vi "LoadConfig.vi"(10 "Path":string, 11 "PN":string) -> (3 "Cluster":T1 {"Screw 2" items=["0", "1", "2", "3", "4", "5", "6", "7", "8", "9", "10", "11", "12", "13", "14", "15", "16", "17", "18", "19", "20", "21", "22", "23", "24", "25", "26", "27", "28", "29", "30"]; "M6_Camera" items=["0", "1", "2", "3", "4", "5", "6", "7", "8", "9", "10", "11", "12", "13", "14", "15", "16", "17", "18", "19", "20", "21", "22", "23", "24", "25", "26", "27", "28", "29", "30"]; "L/R" items=["NA", "RHC-VAC", "RHD-HVAC", "LHD-VAC", "LHD-HVAC", ""]})   [LabVIEW 2020]
uses:
  NewPNConfig.ctl
  <vilib>/Utility/config.llb/Read Key (String).vi
  <vilib>/Utility/config.llb/Read Key (I32).vi
  <vilib>/Utility/config.llb/NI_LVConfig.lvlib
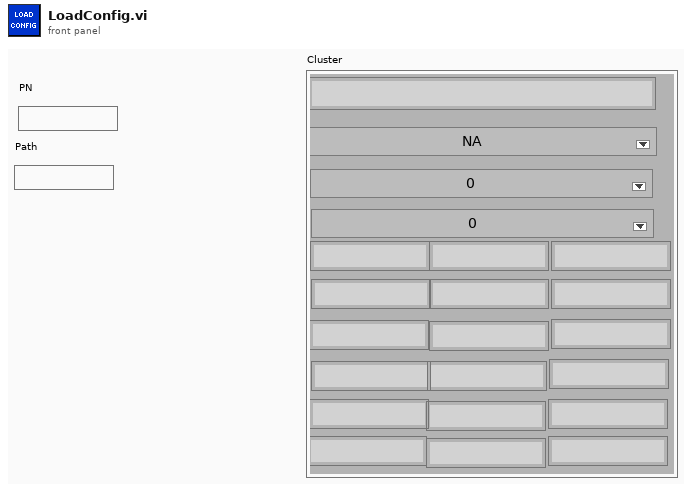
[diagram p1: front panel]
types:
  T1 = typedef "NewPNConfig.ctl" = cluster{"L/R":u8, "PN":string, "M6_Camera":u16, "Screw 2":u16, "Scanner3_1":string, "Scanner3_2":string, "Scanner7_1":string, "Scanner9_1":string, "Scanner9_2":string, "Scanner11_1":string, "Scanner16_1":string, "Scanner19_1":string, "Scanner3_3":string, "Scanner7_2":string, "Scanner7_3":string, "Scanner9_3":string, "Scanner11_2":string, "Scanner11_3":string, "Scanner16_2":string, "Scanner16_3":string, "Scanner19_2":string, "Scanner19_3":string}
  T2 = typedef "NI_LVConfig.lvlib/Config Data RefNum.ctl" = refnum<k1>
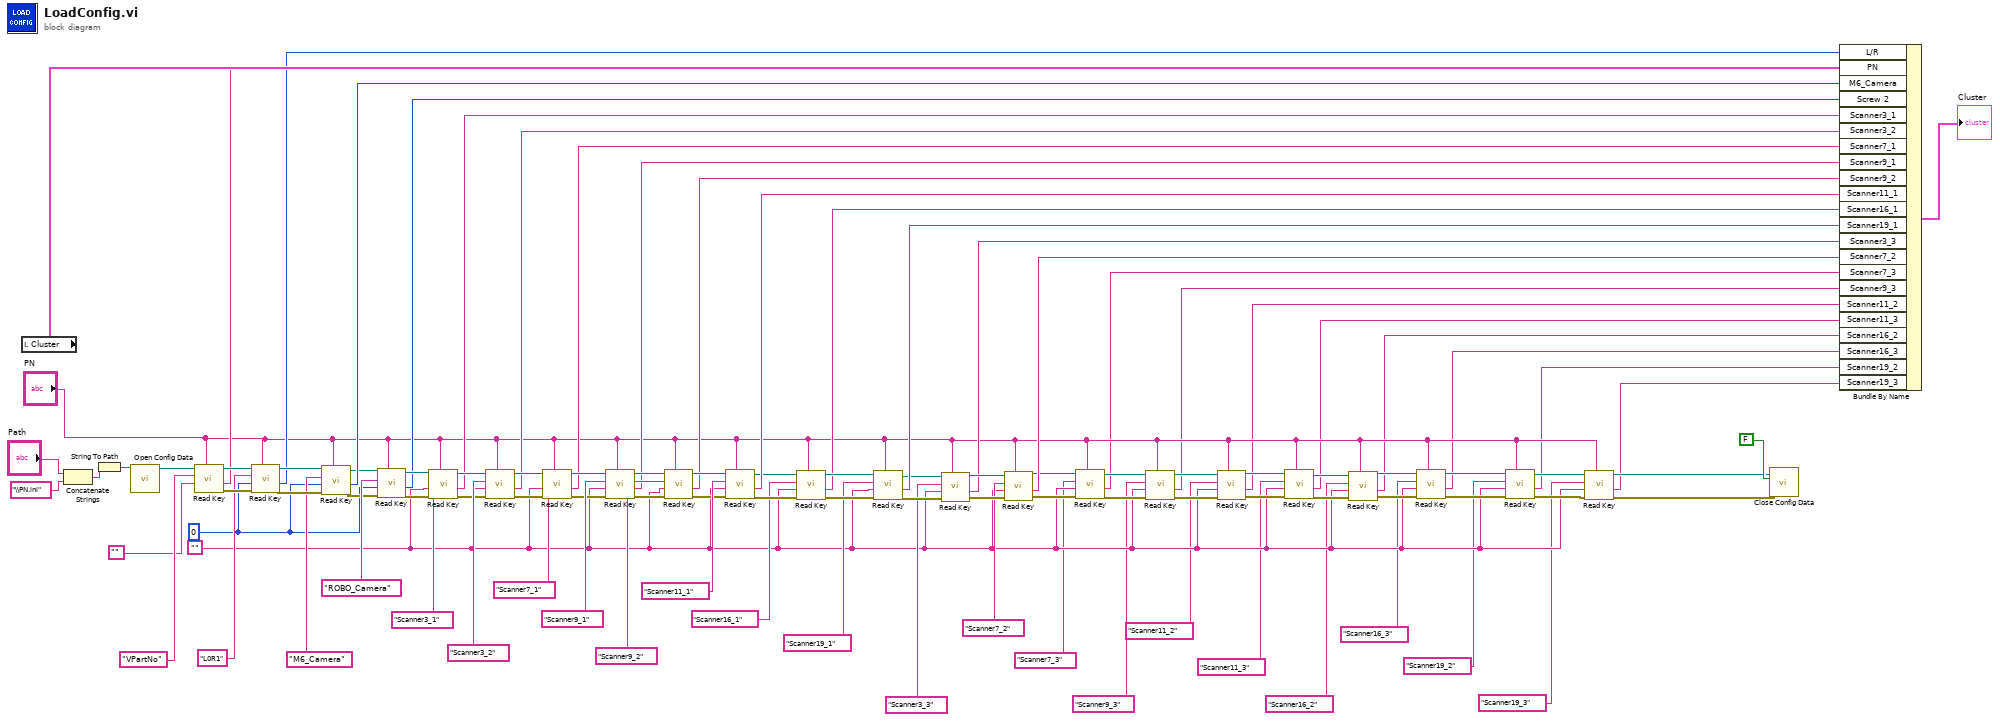
[diagram p0: block diagram]
diagram:
  w17 = ""
  w60 = 0
  n1 = local read "Cluster"() -> (w100:T1)
  n2 = Concatenate Strings("Path", "\\PN.ini") -> (w86:string)
  n3 = String To Path(string=w86) -> (path=w85:path)
  n4 = call <vilib>:"Open Config Data.vi"("configuration file path"=w85) -> ("refnum"=w96:T2)  [unwired: 8 in, 2 out]
  n5 = call-poly <vilib>:"Read Key.vi"("section"="PN", "default value"="", "key"="VPartNo", "refnum"=w96) -> ("error out"=w94:errorcluster, "value"=w89:string, "refnum out"=w98:T2)  [unwired: 4 in, 1 out]
  n6 = call-poly <vilib>:"Read Key.vi"("section"="PN", "error in (no error)"=w94, "default value"=w60, "key"="L0R1", "refnum"=w98) -> ("error out"=w95:errorcluster, "value"=w90:i32, "refnum out"=w97:T2)  [unwired: 3 in, 1 out]
  n7 = call-poly <vilib>:"Read Key.vi"("section"="PN", "error in (no error)"=w95, "default value"=w60, "key"="M6_Camera", "refnum"=w97) -> ("error out"=w68:errorcluster, "value"=w91:i32, "refnum out"=w67:T2)  [unwired: 3 in, 1 out]
  n8 = call-poly <vilib>:"Read Key.vi"("section"="PN", "error in (no error)"=w68, "default value"=w60, "key"="ROBO_Camera", "refnum"=w67) -> ("error out"=w69:errorcluster, "value"=w59:i32, "refnum out"=w66:T2)  [unwired: 3 in, 1 out]
  n9 = call-poly <vilib>:"Read Key.vi"("section"="PN", "error in (no error)"=w69, "default value"=w17, "key"="Scanner3_1", "refnum"=w66) -> ("error out"=w70:errorcluster, "value"=w58:string, "refnum out"=w65:T2)  [unwired: 3 in, 1 out]
  n10 = call-poly <vilib>:"Read Key.vi"("section"="PN", "error in (no error)"=w70, "default value"=w17, "key"="Scanner3_2", "refnum"=w65) -> ("error out"=w71:errorcluster, "value"=w57:string, "refnum out"=w64:T2)  [unwired: 3 in, 1 out]
  n11 = call-poly <vilib>:"Read Key.vi"("section"="PN", "error in (no error)"=w71, "default value"=w17, "key"="Scanner7_1", "refnum"=w64) -> ("error out"=w72:errorcluster, "value"=w56:string, "refnum out"=w63:T2)  [unwired: 3 in, 1 out]
  n12 = call-poly <vilib>:"Read Key.vi"("section"="PN", "error in (no error)"=w72, "default value"=w17, "key"="Scanner9_1", "refnum"=w63) -> ("error out"=w73:errorcluster, "value"=w55:string, "refnum out"=w62:T2)  [unwired: 3 in, 1 out]
  n13 = call-poly <vilib>:"Read Key.vi"("section"="PN", "error in (no error)"=w73, "default value"=w17, "key"="Scanner9_2", "refnum"=w62) -> ("error out"=w74:errorcluster, "value"=w54:string, "refnum out"=w61:T2)  [unwired: 3 in, 1 out]
  n14 = call-poly <vilib>:"Read Key.vi"("section"="PN", "error in (no error)"=w74, "default value"=w17, "key"="Scanner11_1", "refnum"=w61) -> ("error out"=w51:errorcluster, "value"=w53:string, "refnum out"=w52:T2)  [unwired: 3 in, 1 out]
  n15 = call-poly <vilib>:"Read Key.vi"("section"="PN", "error in (no error)"=w51, "default value"=w17, "key"="Scanner16_1", "refnum"=w52) -> ("error out"=w50:errorcluster, "value"=w48:string, "refnum out"=w49:T2)  [unwired: 3 in, 1 out]
  n16 = call-poly <vilib>:"Read Key.vi"("section"="PN", "error in (no error)"=w50, "default value"=w17, "key"="Scanner19_1", "refnum"=w49) -> ("error out"=w43:errorcluster, "value"=w47:string, "refnum out"=w44:T2)  [unwired: 3 in, 1 out]
  n17 = call-poly <vilib>:"Read Key.vi"("section"="PN", "error in (no error)"=w43, "default value"=w17, "key"="Scanner3_3", "refnum"=w44) -> ("error out"=w41:errorcluster, "value"=w39:string, "refnum out"=w40:T2)  [unwired: 3 in, 1 out]
  n18 = call-poly <vilib>:"Read Key.vi"("section"="PN", "error in (no error)"=w41, "default value"=w17, "key"="Scanner7_2", "refnum"=w40) -> ("error out"=w18:errorcluster, "value"=w37:string, "refnum out"=w27:T2)  [unwired: 3 in, 1 out]
  n19 = call-poly <vilib>:"Read Key.vi"("section"="PN", "error in (no error)"=w18, "default value"=w17, "key"="Scanner7_3", "refnum"=w27) -> ("error out"=w19:errorcluster, "value"=w15:string, "refnum out"=w28:T2)  [unwired: 3 in, 1 out]
  n20 = call-poly <vilib>:"Read Key.vi"("section"="PN", "error in (no error)"=w19, "default value"=w17, "key"="Scanner9_3", "refnum"=w28) -> ("error out"=w20:errorcluster, "value"=w13:string, "refnum out"=w29:T2)  [unwired: 3 in, 1 out]
  n21 = call-poly <vilib>:"Read Key.vi"("section"="PN", "error in (no error)"=w20, "default value"=w17, "key"="Scanner11_2", "refnum"=w29) -> ("error out"=w21:errorcluster, "value"=w12:string, "refnum out"=w30:T2)  [unwired: 3 in, 1 out]
  n22 = call-poly <vilib>:"Read Key.vi"("section"="PN", "error in (no error)"=w21, "default value"=w17, "key"="Scanner11_3", "refnum"=w30) -> ("error out"=w22:errorcluster, "value"=w9:string, "refnum out"=w31:T2)  [unwired: 3 in, 1 out]
  n23 = call-poly <vilib>:"Read Key.vi"("section"="PN", "error in (no error)"=w22, "default value"=w17, "key"="Scanner16_2", "refnum"=w31) -> ("error out"=w23:errorcluster, "value"=w8:string, "refnum out"=w32:T2)  [unwired: 3 in, 1 out]
  n24 = call-poly <vilib>:"Read Key.vi"("section"="PN", "error in (no error)"=w23, "default value"=w17, "key"="Scanner16_3", "refnum"=w32) -> ("error out"=w24:errorcluster, "value"=w5:string, "refnum out"=w33:T2)  [unwired: 3 in, 1 out]
  n25 = call-poly <vilib>:"Read Key.vi"("section"="PN", "error in (no error)"=w24, "default value"=w17, "key"="Scanner19_2", "refnum"=w33) -> ("error out"=w25:errorcluster, "value"=w4:string, "refnum out"=w34:T2)  [unwired: 3 in, 1 out]
  n26 = call-poly <vilib>:"Read Key.vi"("section"="PN", "error in (no error)"=w25, "default value"=w17, "key"="Scanner19_3", "refnum"=w34) -> ("error out"=w36:errorcluster, "value"=w1:string, "refnum out"=w35:T2)  [unwired: 3 in, 1 out]
  n27 = call <vilib>:"Close Config Data.vi"("error in (no error)"=w36, "write file if changed (T)"=FALSE, "refnum"=w35) -> ()  [unwired: 7 in, 2 out]
  n28 = Bundle By Name(cluster=w100, "L/R"=w90, "PN"=w89, "M6_Camera"=w91, "Screw 2"=w59, "Scanner3_1"=w58, "Scanner3_2"=w57, "Scanner7_1"=w56, "Scanner9_1"=w55, "Scanner9_2"=w54, "Scanner11_1"=w53, "Scanner16_1"=w48, "Scanner19_1"=w47, "Scanner3_3"=w39, "Scanner7_2"=w37, "Scanner7_3"=w15, "Scanner9_3"=w13, "Scanner11_2"=w12, "Scanner11_3"=w9, "Scanner16_2"=w8, "Scanner16_3"=w5, "Scanner19_2"=w4, "Scanner19_3"=w1) -> (→"Cluster":T1)
